vi "Teleop.vi"(10 "Match Info":T1={"Autonomous Elapsed Seconds"=0.0, "TeleOp Elapsed Seconds"=0.0, "Disabled Elapsed Seconds"=0.0, "Visited Autonomous"=FALSE, "Visited TeleOp"=FALSE, "Visited Disabled"=FALSE, "Autonomous Settings"={"Autonomous Style"=enum."Independent", "VI Refnum"=refnum}}, 11 "Call Context":T2) -> ()   [LabVIEW 2011]
doc: "This VI is called for each TeleOp packet received from the DS where the robot is not disabled. It is often used to read from the joysticks and update I/O or to update setpoints for timed control loops. It should complete and return within 20 milliseconds or it may miss DS packets."
uses:
  <vilib>/Rock Robotics/WPI/DriverStation/WPI_DriverStationDerivedRobotMode.ctl
  <vilib>/Rock Robotics/WPI/DriverStation/WPI_DriverStationMatch Info.ctl
  Robot Global Data.vi
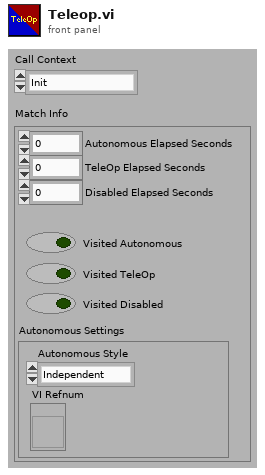
[diagram p1: front panel]
types:
  T1 = typedef "WPI_DriverStationMatch Info.ctl" = cluster{"Autonomous Elapsed Seconds":dbl, "TeleOp Elapsed Seconds":dbl, "Disabled Elapsed Seconds":dbl, "Visited Autonomous":bool, "Visited TeleOp":bool, "Visited Disabled":bool, "Autonomous Settings":cluster{"Autonomous Style":enum16{"Iterative", "Independent"}, "VI Refnum":refnum<vi>}}
  T2 = typedef "WPI_DriverStationDerivedRobotMode.ctl" = enum16{"Init", "Execute", "Stop"}
  T3 = typedef "WPI_MotorControlDeviceRef.ctl" = cluster{"DeviceStatus":errorcluster, "Type":enum16{"PWM", "CAN"}, "PWM":cluster{"Digital Module":T4, "PWM Channel":T5, "DeadBand":T6}, "CAN":cluster{"Device Number":u8, "Control Mode":T7, "Semaphore":T8, "Max Vout":dbl}, "Invert":bool, "TransformRef":T9, "InvTransformRef":T9}
  T4 = typedef "FPGA_TypedefDigitalModule.ctl" = enum16{"Digital Module 1", "Digital Module 2"}
  T5 = typedef "FPGA_DIOPWMChannel.ctl" = enum8{"PWM 1", "PWM 2", "PWM 3", "PWM 4", "PWM 5", "PWM 6", "PWM 7", "PWM 8", "PWM 9", "PWM 10", "Invalid"}
  T6 = typedef "WPI_PWMDeadband.ctl" = cluster{"Name":string, "maxPositivePwm":i32, "minPositivePwm":i32, "centerPwm":i32, "maxNegativePwm":i32, "minNegativePwm":i32, "angularRange":u16}
  T7 = typedef "WPI_CANJaguar_ControlMode.ctl" = enum8{"Percent VBus", "Current", "Speed", "Position", "Voltage"}
  T8 = typedef "Semaphore RefNum" = refnum<k1>
  T9 = typedef "WPI_PWMTransform_ConPane.ctl" = refnum<vi>
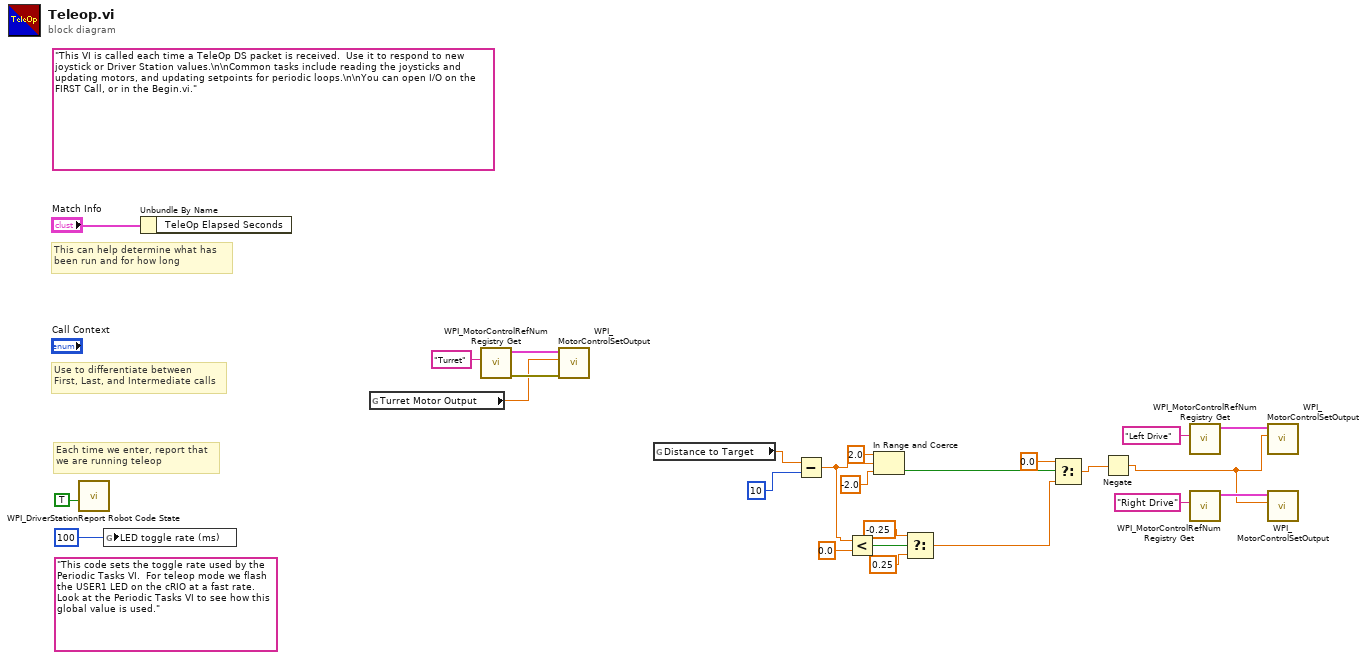
[diagram p0: block diagram]
diagram:
  (unwired) "This code sets the toggle rate used by the Periodic Tasks VI.  For teleop mode we flash the USER1 LED on the cRIO at a fast rate.  Look at the Periodic Tasks VI to see how this global value is used."
  (unwired) "This VI is called each time a TeleOp DS packet is received.  Use it to respond to new joystick or Driver Station values.\n\nCommon tasks include reading the joysticks and updating motors, and updating setpoints for periodic loops.\n\nYou can open I/O on the FIRST Call, or in the Begin.vi."
  # "Each time we enter, report that\nwe are running teleop"
  # "Use to differentiate between\nFirst, Last, and Intermediate calls"
  # "This can help determine what has\nbeen run and for how long"
  n1 = call <vilib>:"WPI_DriverStationReport Robot Code State.vi"("TeleOp"=TRUE ("Autonomous")) -> ()  [unwired: 10 in, 1 out]
  n2 = global write "Robot Global Data.vi" "LED toggle rate (ms)"(u32 100 ("LED ms toggle rate")) -> ()
  n3 = Unbundle By Name("Match Info") -> ()  [unwired: 1 out]
  n4 = global read "Robot Global Data.vi" "Turret Motor Output"() -> (w19:dbl)
  n5 = call <vilib>:"WPI_MotorControlRefNum Registry Get.vi"("refnum name"="Turret") -> ("error out"=w20:errorcluster, "MotorControlDevRef"=w21:T3)  [unwired: 9 in]
  n6 = call <vilib>:"WPI_MotorControlSetOutput.vi"("error in (no error)"=w20, "Output"=w19, "MotorControlDevRef"=w21) -> ()  [unwired: 7 in, 2 out]
  n7 = global read "Robot Global Data.vi" "Distance to Target"() -> (w14:dbl)
  n8 = Subtract(x=w14, y=10) -> (x-y=w7:dbl)
  n9 = Less?(x=w7, y=0.0) -> (x < y?=w6:bool)
  n10 = In Range and Coerce(upper limit=2.0, x=w7, lower limit=-2.0) -> (In Range?=w10:bool)  [unwired: 1 out]
  n11 = Select(t=-0.25, s=w6, f=0.25) -> (s? t:f=w3:dbl)
  n12 = Select(t=0.0, s=w10, f=w3) -> (s? t:f=w2:dbl)
  n13 = Negate(x=w2) -> (-x=w1:dbl)
  n14 = call <vilib>:"WPI_MotorControlRefNum Registry Get.vi"("refnum name"="Left Drive") -> ("MotorControlDevRef"=w18:T3)  [unwired: 9 in, 1 out]
  n15 = call <vilib>:"WPI_MotorControlRefNum Registry Get.vi"("refnum name"="Right Drive") -> ("MotorControlDevRef"=w15:T3)  [unwired: 9 in, 1 out]
  n16 = call <vilib>:"WPI_MotorControlSetOutput.vi"("Output"=w1, "MotorControlDevRef"=w18) -> ()  [unwired: 8 in, 2 out]
  n17 = call <vilib>:"WPI_MotorControlSetOutput.vi"("Output"=w1, "MotorControlDevRef"=w15) -> ()  [unwired: 8 in, 2 out]
